vi "超标留样全局.vi"() -> ()   [LabVIEW 2016, in "超标留样集成.lvlib" / "ESTD1200.lvlib"]
uses:
  ESTD1200.lvlib
  <vilib>/Plasmionique/MB Master/MB_Master/MB_Master.lvclass
panel:
  out "传感器实时浓度":T1
  out "状态告警区":T2 {"告警代码" items=["无告警", "通讯异常(采样器与工控机通讯)", "滑台电机异常(过温/过流)", "蠕动泵异常(过温/过流)", "转盘电机异常(过温/过流)", "编码器异常", "转盘原点传感器异常", "滑台原点传感器异常", "冰箱温度异常", "冰箱通讯异常", "门禁锁异常", "串口屏通讯异常", "SD卡异常告警", "Flash异常告警(W25Q32)", "留样失败", "瓶满告警", "复位异常"]; "采样模式" items=["定时采样", "外控采样", "时间等比", "流量等比", "液位等比"]; "当前进程" items=["待机", "电机复位", "采样瓶转到采样区", "采样瓶排空", "采样泵管润洗", "采样瓶再排空", "采样", "采样泵反转排空管路", "取样瓶转到取样区"]}
  out "系统设置区":T3
  out "采样模式区":T4 {"采样模式" items=["定时采样", "外控采样", "时间等比", "流量等比", "液位等比"]}
  out "采样状态区":T5 {"当前进程" items=["待机", "电机复位", "采样瓶转到采样区", "采样瓶排空", "采样泵管润洗", "采样瓶再排空", "采样", "采样泵反转排空管路", "取样瓶转到取样区"]; "采样模式" items=["定时采样", "外控采样", "时间等比", "流量等比", "液位等比"]; "采样器状态" items=["空闲", "忙碌"]}
  out "MB session in":refnum<class "MB_Master.lvclass">
  out "通讯":bool
  in  "当前瓶号":u16
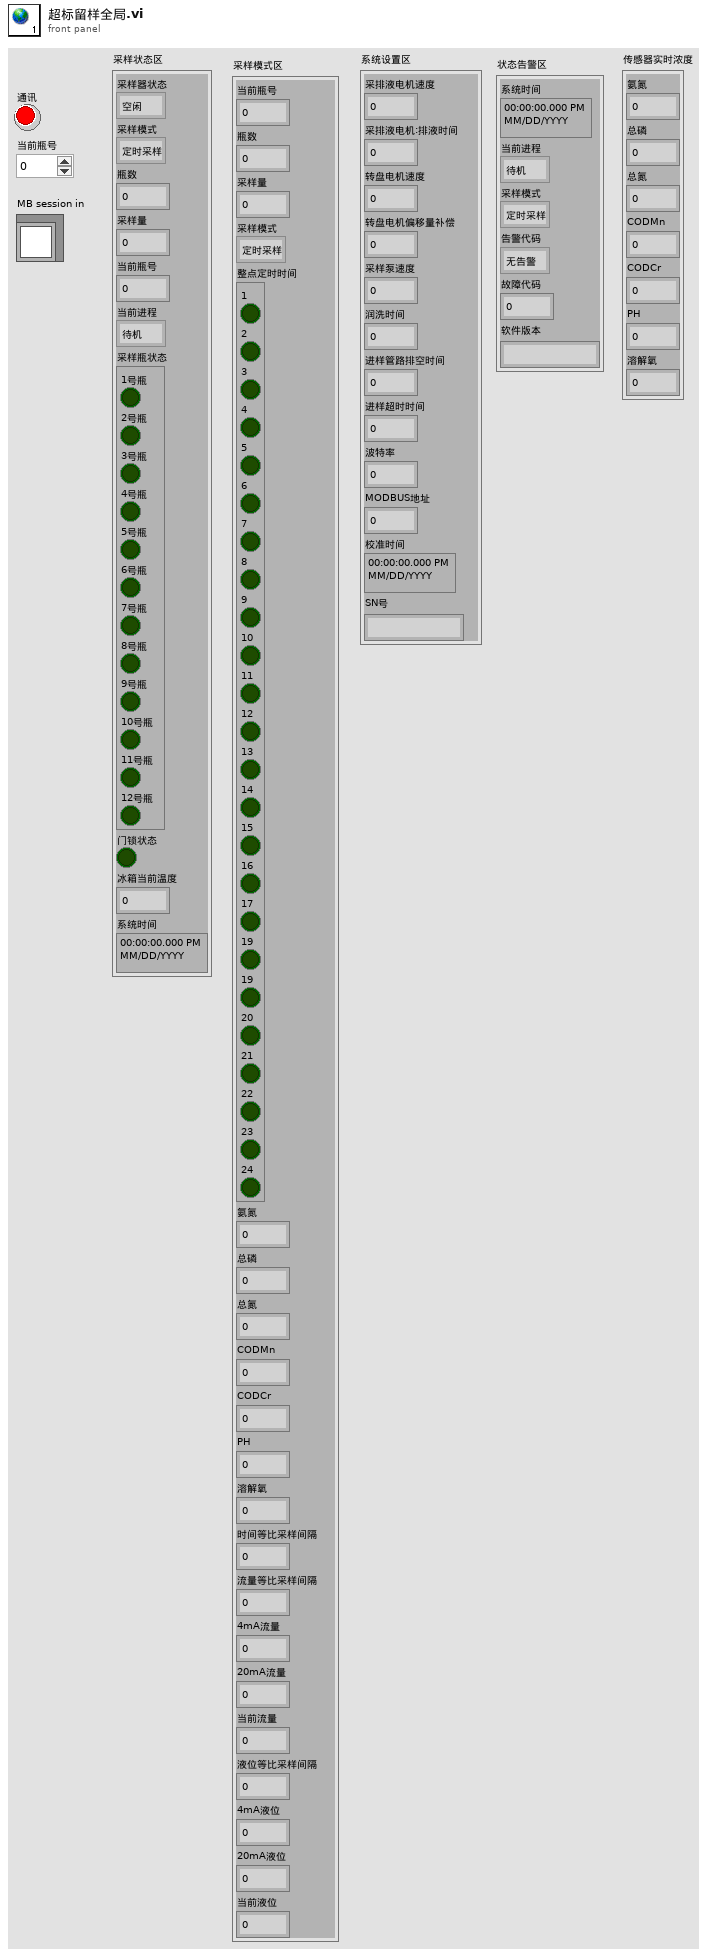
[diagram p1: front panel]
types:
  T1 = cluster{"氨氮":sgl, "总磷":sgl, "总氮":sgl, "CODMn":sgl, "CODCr":sgl, "PH":sgl, "溶解氧":sgl}
  T2 = cluster{"系统时间":timestamp, "当前进程":u16, "采样模式":u16, "告警代码":u16, "故障代码":u16, "软件版本":string}
  T3 = cluster{"采排液电机速度":u16, "采排液电机:排液时间":u16, "转盘电机速度":u16, "转盘电机偏移量补偿":i16, "采样泵速度":u16, "润洗时间":u16, "进样管路排空时间":u16, "进样超时时间":u16, "波特率":u16, "MODBUS地址":u16, "校准时间":timestamp, "SN号":string}
  T4 = cluster{"当前瓶号":u16, "瓶数":u16, "采样量":u16, "采样模式":u16, "整点定时时间":cluster{"1":bool, "2":bool, "3":bool, "4":bool, "5":bool, "6":bool, "7":bool, "8":bool, "9":bool, "10":bool, "11":bool, "12":bool, "13":bool, "14":bool, "15":bool, "16":bool, "17":bool, "19":bool, "19":bool, "20":bool, "21":bool, "22":bool, "23":bool, "24":bool}, "氨氮":sgl, "总磷":sgl, "总氮":sgl, "CODMn":sgl, "CODCr":sgl, "PH":sgl, "溶解氧":sgl, "时间等比采样间隔":u16, "流量等比采样间隔":sgl, "4mA流量":sgl, "20mA流量":sgl, "当前流量":sgl, "液位等比采样间隔":sgl, "4mA液位":sgl, "20mA液位":sgl, "当前液位":sgl}
  T5 = cluster{"采样器状态":u16, "采样模式":u16, "瓶数":u16, "采样量":u16, "当前瓶号":u16, "当前进程":u16, "采样瓶状态":cluster{"1号瓶":bool, "2号瓶":bool, "3号瓶":bool, "4号瓶":bool, "5号瓶":bool, "6号瓶":bool, "7号瓶":bool, "8号瓶":bool, "9号瓶":bool, "10号瓶":bool, "11号瓶":bool, "12号瓶":bool}, "门锁状态":bool, "冰箱当前温度":sgl, "系统时间":timestamp}
diagram:
